vi "Tree to KVP.vi"(10 "Variant Tree":variant) -> (2 "KVP":variant)   [LabVIEW 2013, in "OpenVariant.lvlib"]
uses:
  OpenVariant.lvlib
  TypeDescriptor/TypeDescriptor_GetType.vi
  <vilib>/Utility/VariantDataType/GetTypeInfo.vi
  Conversions/OpenConvert.lvlib
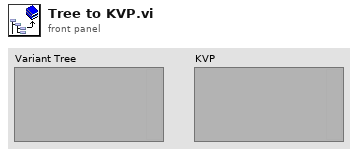
[diagram p1: front panel]
types:
  T1 = typedef "VariantType.lvlib/Type.ctl" = enum8{"Invalid Type", "Void", "I8", "I16", "I32", "I64", "U8", "U16", "U32", "U64", "Single Float", "Double Float", "Extended Float", "Single Complex", "Double Complex", "Extended Complex", "Enum U8", "Enum U16", "Enum U32", "Enum U64", "Single Float With Unit", "Double Float With Unit", "Extended Float With Unit", "Single Complex with Unit", "Double Complex with Unit", "Extended Complex with Unit", "Boolean", "String", "Path", "Picture", "Tag", "Array", "Cluster", "Variant", "LV Variant", "Waveform", "Timestamp", "Digital Waveform", "Digital Data", "ExpressData", "Refnum", "External Data", "VI", "Poly VI", "LabVIEW Class Instance", "Fixed Point"}
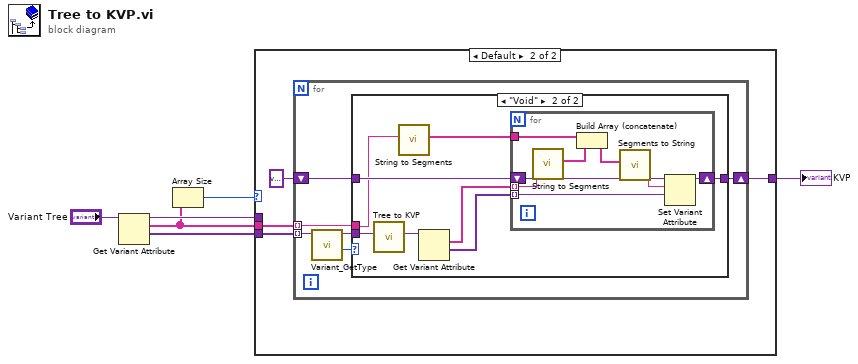
[diagram p0: block diagram]
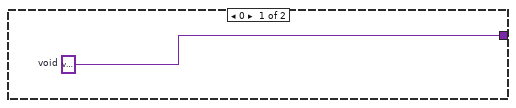
[diagram p2: hidden frame]
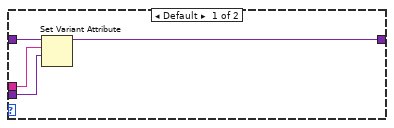
[diagram p3: hidden frame]
diagram:
  n1 = Get Variant Attribute(Variant="Variant Tree") -> (duplicate Variant=w6:variant, names=w3:string[], values=w2:variant[])  [unwired: 3 in, 1 out]
  n2 = Array Size(array=w3) -> (size(s)=w4:i32)
  n3 = case shown="Default" w4 {
    tunnel: w2 -> [_ w11]
    tunnel: w3 -> [_ w10]
    tunnel: [w7 w8] -> w1
    tunnel: w6 -> [_ _]
    frame 0 {
      w7 = variant  # void
    }
    frame Default {
      n4 = for {
        tunnel: w11 -> [w17] mode=indexing
        tunnel: w10 -> [w14] mode=indexing
        shift-right: [w12] -> w8
        shift-left: variant ("duplicate variant") -> [w13]
        n5 = call "Variant_GetType.vi"("Variant"=w17) -> ("LV Type Enum"=w15:T1, "Variant dup"=w16:variant)  [unwired: 8 in, 1 out]
        n6 = case shown="\"Void\"" w15 {
          tunnel: w16 -> [w19 w29]
          tunnel: w14 -> [w20 w23]
          tunnel: w13 -> [w21 w27]
          tunnel: [w18 w26] -> w12
          frame Default {
            n7 = Set Variant Attribute(Variant=w21, name=w20, value=w19) -> (Variant out=w18:variant)  [unwired: 1 in, 2 out]
          }
          frame "Void" {
            n8 = call "Tree to KVP.vi"("Variant Tree"=w29) -> ("KVP"=w28:variant)  [unwired: 10 in]
            n9 = call "String to Segments.vi"("String"=w23) -> ("Segments"=w22:string[])  [unwired: 9 in, 1 out]
            n10 = Get Variant Attribute(Variant=w28) -> (names=w25:string[], values=w24:variant[])  [unwired: 3 in, 2 out]
            n11 = for {
              tunnel: w25 -> [w33] mode=indexing
              tunnel: w24 -> [w35] mode=indexing
              shift-right: [w36] -> w26
              shift-left: w27 -> [w37]
              tunnel: w22 -> [w32]
              n12 = call "String to Segments.vi"("String"=w33) -> ("Segments"=w31:string[])  [unwired: 9 in, 1 out]
              n13 = Build Array (concatenate)(w32, w31) -> (w30:string[])
              n14 = call "Segments to String.vi"("Segments"=w30) -> ("String"=w34:string)  [unwired: 10 in]
              n15 = Set Variant Attribute(Variant=w37, name=w34, value=w35) -> (Variant out=w36:variant)  [unwired: 1 in, 2 out]
            }
          }
        }
      }
    }
  }
  "KVP" <- w1
